vi "_CSMObj-Release CSM.vi"(8 "Error In":errorcluster caption="error in (no error)", 11 "CSMQ In":T1={"info"={"Module Name"="", "Requested Name"="", "Group Name"="", "Mode"=enum."Stand Alone", "Allowed Messages"=[]}, "Refs"={"WatchDogQ"=refnum, "CSMDataDVR"=refnum, "Queue"={"HPriorityQ"=refnum, "LowPriorityQ"=refnum}, "GroupDataDVR"=refnum, "TagMap"=refnum, "ExitEvent"=refnum, "NewStateEvent"=refnum, "StatusEvent"=refnum, "InterruptEvent"=refnum}}) -> (0 "error out":errorcluster, 1 "Group Release?":bool, 3 "CSMQ Out":T1={"info"={"Module Name"="", "Requested Name"="", "Group Name"="", "Mode"=enum."Stand Alone", "Allowed Messages"=[]}, "Refs"={"WatchDogQ"=refnum, "CSMDataDVR"=refnum, "Queue"={"HPriorityQ"=refnum, "LowPriorityQ"=refnum}, "GroupDataDVR"=refnum, "TagMap"=refnum, "ExitEvent"=refnum, "NewStateEvent"=refnum, "StatusEvent"=refnum, "InterruptEvent"=refnum}})   [LabVIEW 2017, in "Communicable State Machine.lvlib"]
uses:
  Communicable State Machine.lvlib
  _CSMObj.ctl
  _CSMObj-Info.ctl
  Typedef/_CSM_MODE.ctl
  _CSMObj-Refs.ctl
  _CSMObj-Data.ctl
  Priority Queue/Priority Queue.ctl
  Typedef/_Cross CSM State Data.ctl
  Typedef/_CSM_MSG_TYPE.ctl
  Typedef/_Cross CSM State Response.ctl
  Typedef/_CSM_Response Source Message.ctl
  Priority Queue/def-Data(LowPRI-Q).ctl
  _CSMObj-ModeData.ctl
  Typedef/_CSM Status Change Event Data.ctl
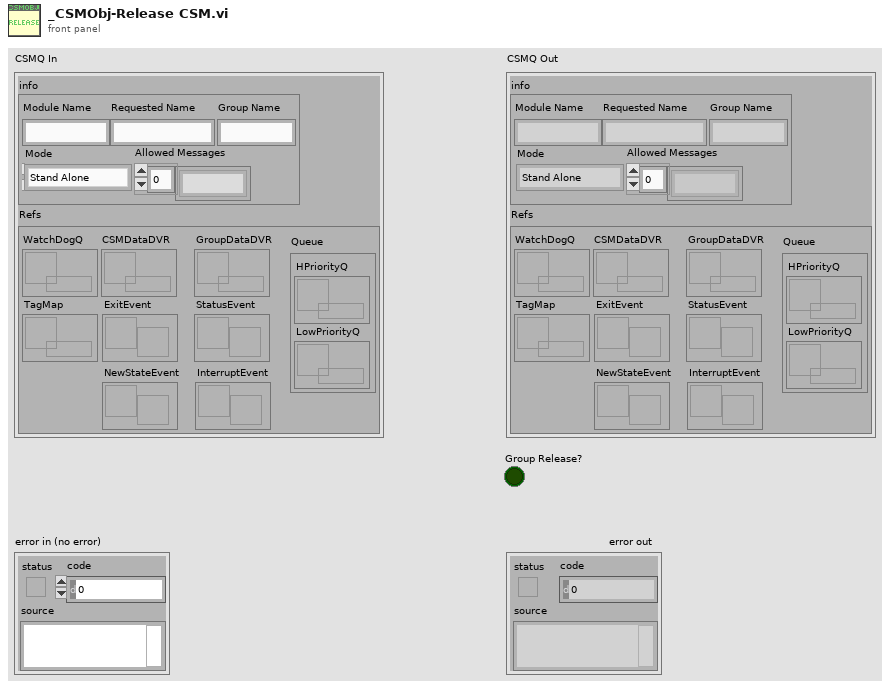
[diagram p1: front panel]
types:
  T1 = typedef "Communicable State Machine.lvlib/_CSMObj.ctl" = cluster{"info":T2, "Refs":T4}
  T2 = typedef "Communicable State Machine.lvlib/_CSMObj-Info.ctl" = cluster{"Module Name":string, "Requested Name":string, "Group Name":string, "Mode":T3, "Allowed Messages":string[]}
  T3 = typedef "Communicable State Machine.lvlib/_CSM_MODE.ctl" = enum16{"Not Exist", "Stand Alone", "CSM", "Worker", "Worker Agent", "Chain Node", "Chain"}
  T4 = typedef "Communicable State Machine.lvlib/_CSMObj-Refs.ctl" = cluster{"WatchDogQ":refnum<queue>, "CSMDataDVR":refnum<data-value>, "Queue":T5, "GroupDataDVR":refnum<data-value>, "TagMap":refnum<data-value>, "ExitEvent":refnum<user-event>, "NewStateEvent":refnum<user-event>, "StatusEvent":refnum<user-event>, "InterruptEvent":refnum<user-event>}
  T5 = typedef "Communicable State Machine.lvlib/Priority Queue.ctl" = cluster{"HPriorityQ":refnum<queue>, "LowPriorityQ":refnum<queue>}
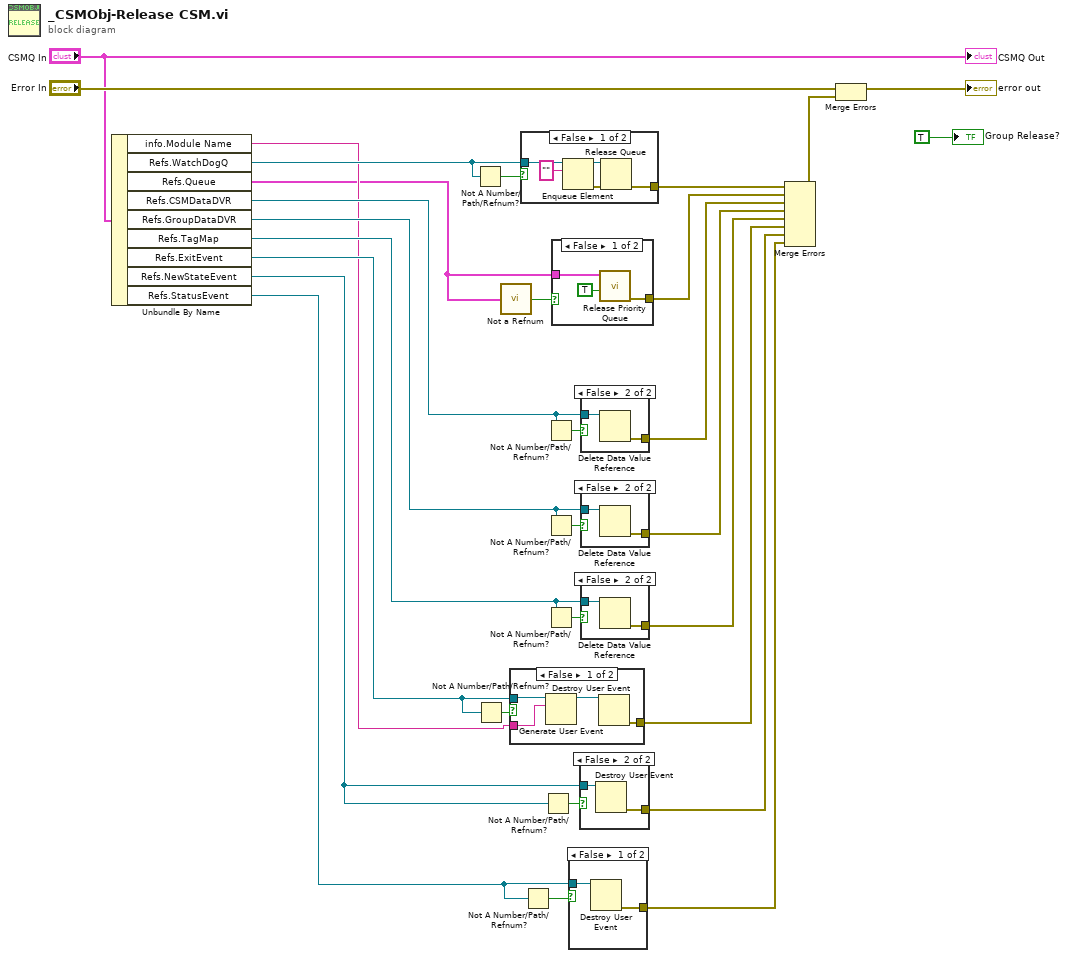
[diagram p0: block diagram]
diagram:
  n1 = Unbundle By Name("CSMQ In") -> ("info.Module Name"=w4:string, "Refs.WatchDogQ"=w16:refnum<queue>, "Refs.Queue"=w1:T5, "Refs.CSMDataDVR"=w14:refnum<data-value>, "Refs.GroupDataDVR"=w12:refnum<data-value>, "Refs.TagMap"=w9:refnum<data-value>, "Refs.ExitEvent"=w5:refnum<user-event>, "Refs.NewStateEvent"=w25:refnum<user-event>, "Refs.StatusEvent"=w26:refnum<user-event>)
  n2 = Not A Number/Path/Refnum?(number/path/refnum=w16) -> (NaN/Path/Refnum?=w18:bool)
  n3 = Not A Number/Path/Refnum?(number/path/refnum=w5) -> (NaN/Path/Refnum?=w7:bool)
  n4 = call "Not a Refnum.vi"("Priority Queue.lvclass"=w1) -> ("NaN/Path/Refnum?"=w3:bool)  [unwired: 4 in]
  n5 = case shown="False" w7 {
    tunnel: [w34 _] -> w6
    tunnel: w5 -> [w33 _]
    tunnel: w4 -> [w31 _]
    frame False {
      n6 = Generate User Event(user event=w33, event data cluster=w31) -> (user event out=w32:refnum<user-event>)  [unwired: 2 in, 1 out]
      n7 = Destroy User Event(user event=w32) -> (error out=w34:errorcluster)  [unwired: 1 in]
    }
    frame True {
    }
  }
  n8 = case shown="False" w18 {
    tunnel: [w39 _] -> w15
    tunnel: w16 -> [w38 _]
    frame False {
      n9 = Enqueue Element(queue=w38, element="") -> (queue out=w37:refnum<queue>, error out=w35:errorcluster)  [unwired: 2 in, 1 out]
      n10 = Release Queue(queue=w37, error in (no error)=w35) -> (error out=w39:errorcluster)  [unwired: 1 in, 2 out]
    }
    frame True {
    }
  }
  n11 = Not A Number/Path/Refnum?(number/path/refnum=w26) -> (NaN/Path/Refnum?=w21:bool)
  n12 = Not A Number/Path/Refnum?(number/path/refnum=w25) -> (NaN/Path/Refnum?=w20:bool)
  n13 = Not A Number/Path/Refnum?(number/path/refnum=w14) -> (NaN/Path/Refnum?=w19:bool)
  n14 = Not A Number/Path/Refnum?(number/path/refnum=w12) -> (NaN/Path/Refnum?=w13:bool)
  n15 = Not A Number/Path/Refnum?(number/path/refnum=w9) -> (NaN/Path/Refnum?=w10:bool)
  n16 = case shown="False" w3 {
    tunnel: w1 -> [w42 _]
    tunnel: [w40 _] -> w2
    frame False {
      n17 = call "Release Priority Queue.vi"("Force Destroy? (F)"=TRUE ("force destroy? (F)"), "Priority Queue"=w42) -> ("error out"=w40:errorcluster)  [unwired: 9 in]
    }
    frame True {
    }
  }
  n18 = case shown="False" w21 {
    tunnel: [w44 _] -> w22
    tunnel: w26 -> [w43 _]
    frame False {
      n19 = Destroy User Event(user event=w43) -> (error out=w44:errorcluster)  [unwired: 1 in]
    }
    frame True {
    }
  }
  n20 = case shown="False" w20 {
    tunnel: [_ w46] -> w23
    tunnel: w25 -> [_ w45]
    frame True {
    }
    frame False {
      n21 = Destroy User Event(user event=w45) -> (error out=w46:errorcluster)  [unwired: 1 in]
    }
  }
  n22 = case shown="False" w19 {
    tunnel: [_ w48] -> w24
    tunnel: w14 -> [_ w47]
    frame True {
    }
    frame False {
      n23 = Delete Data Value Reference(data value reference=w47) -> (error out=w48:errorcluster)  [unwired: 1 in, 1 out]
    }
  }
  n24 = case shown="False" w13 {
    tunnel: [_ w50] -> w11
    tunnel: w12 -> [_ w49]
    frame True {
    }
    frame False {
      n25 = Delete Data Value Reference(data value reference=w49) -> (error out=w50:errorcluster)  [unwired: 1 in, 1 out]
    }
  }
  n26 = case shown="False" w10 {
    tunnel: [_ w52] -> w8
    tunnel: w9 -> [_ w51]
    frame True {
    }
    frame False {
      n27 = Delete Data Value Reference(data value reference=w51) -> (error out=w52:errorcluster)  [unwired: 1 in, 1 out]
    }
  }
  n28 = Merge Errors(w15, w2, w24, w11, w8, w6, w23, w22) -> (w28:errorcluster)
  n29 = Merge Errors("Error In", w28) -> (→"error out":errorcluster)
  "CSMQ Out" <- "CSMQ In"
  "Group Release?" <- TRUE
